vi "MGI SRS Table Settings.vi"(7 "Command":T1, 8 "Error In":errorcluster, 10 "MCLB Info In":T2, 11 "Graph/Chart Ref":refnum<vi>) -> (0 "Error Out":errorcluster, 2 "MCLB Info Out":T2)   [LabVIEW 2020]
doc: "Populates the Table Settings cluster with values from the Table of the specified Refnum.\n\nNote: Only the columns that have header strings are saved.\n\nAuthored by Shawn Walpole\nsupport@mooregoodideas.com\nwww.mooregoodideas.com\n\nCopyright (c) 2010, Moore Good Ideas, Inc.\n\nAll rights reserved.\n\nRedistribution and use in source and binary forms, with or without modification, are permitted provided that the following conditions are met:\n\n * Redistributions of source code must retain the above copyright notice, this list of conditions and the following disclaimer.\n * Redistributions in binary form must reproduce the above copyright notice, this list of conditions and the following disclaimer in the documentation and/or other materials provided with the distribution.\n * Neither the name of Moore Good Ideas, Inc. nor the names of its contributors may be used to endorse or promote products derived from this software without specific prior written permission.\n\nTHIS SOFTWARE IS PROVIDED BY THE COPYRIGHT HOLDERS AND CONTRIBUTORS \"AS IS\" AND ANY EXPRESS OR IMPLIED WARRANTIES, INCLUDING, BUT NOT LIMITED TO, THE IMPLIED WARRANTIES OF MERCHANTABILITY AND FITNESS FOR A PARTICULAR PURPOSE ARE DISCLAIMED. IN NO EVENT SHALL THE COPYRIGHT OWNER OR CONTRIBUTORS BE LIABLE FOR ANY DIRECT, INDIRECT, INCIDENTAL, SPECIAL, EXEMPLARY, OR CONSEQUENTIAL DAMAGES (INCLUDING, BUT NOT LIMITED TO, PROCUREMENT OF SUBSTITUTE GOODS OR SERVICES; LOSS OF USE, DATA, OR PROFITS; OR BUSINESS INTERRUPTION) HOWEVER CAUSED AND ON ANY THEORY OF LIABILITY, WHETHER IN CONTRACT, STRICT LIABILITY, OR TORT (INCLUDING NEGLIGENCE OR OTHERWISE) ARISING IN ANY WAY OUT OF THE USE OF THIS SOFTWARE, EVEN IF ADVISED OF THE POSSIBILITY OF SUCH DAMAGE."
uses:
  <userlib>/_MGI/Application Control/MGI Save & Restore Settings/MGI SRS Command Enum.ctl
  <userlib>/_MGI/Application Control/MGI Save & Restore Settings/MGI SRS MCLB Setting Cluster.ctl
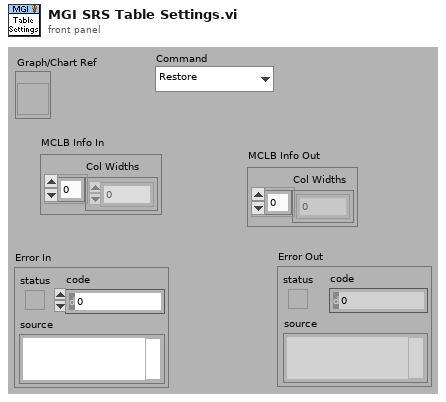
[diagram p1: front panel]
types:
  T1 = typedef "MGI SRS Command Enum.ctl" = enum16{"Restore", "Save"}
  T2 = typedef "MGI SRS MCLB Setting Cluster.ctl" = cluster{"Col Widths":i32[]}
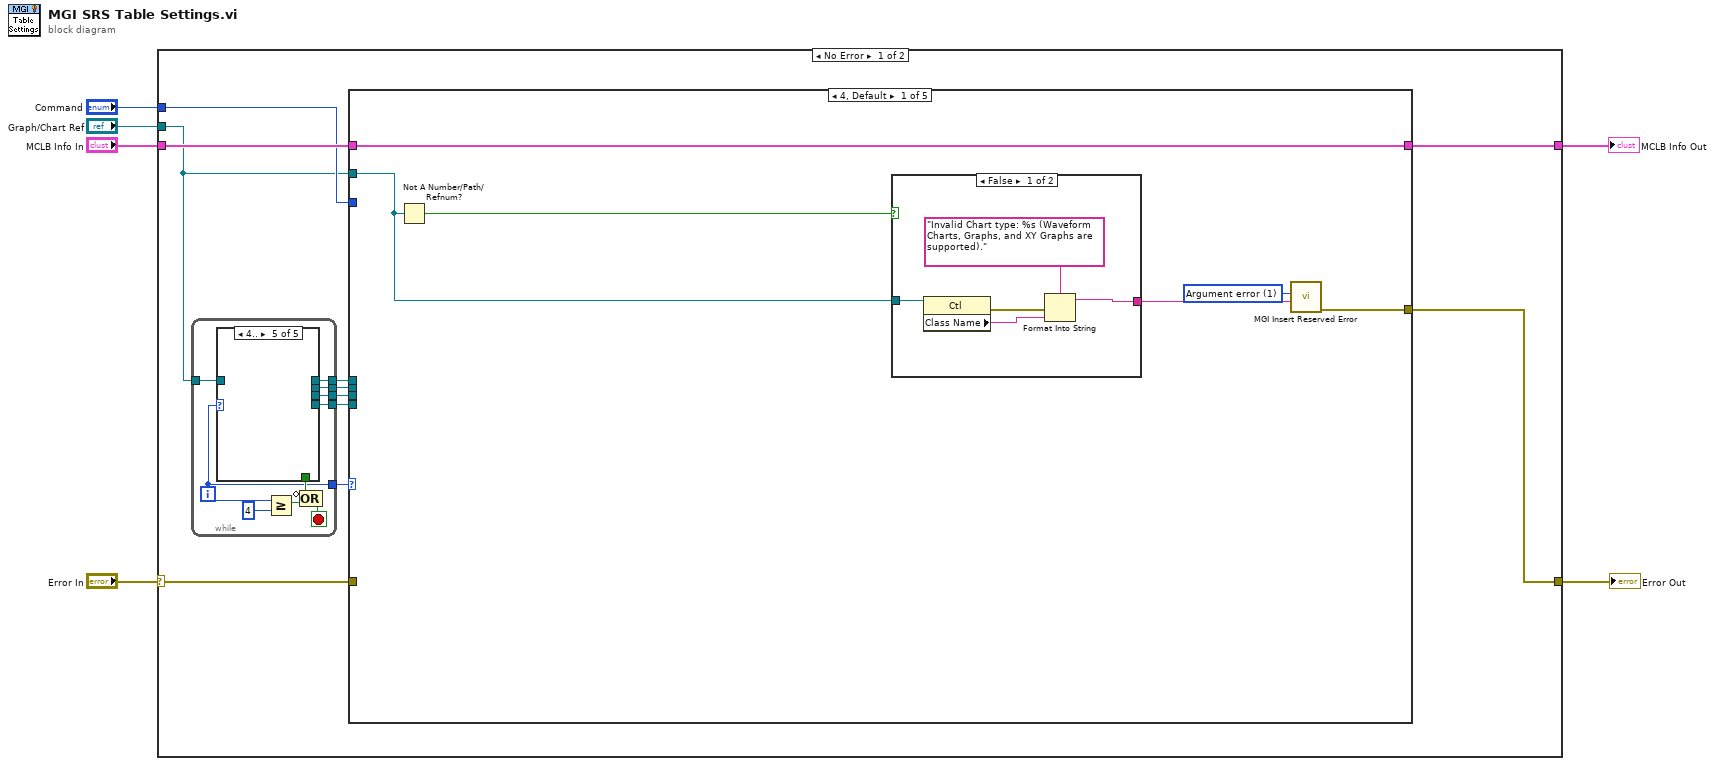
[diagram p0: block diagram]
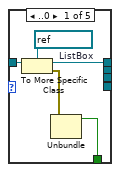
[diagram p2: hidden frame]
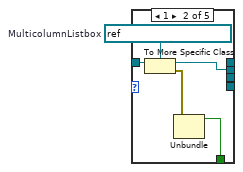
[diagram p3: hidden frame]
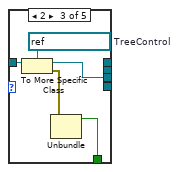
[diagram p4: hidden frame]
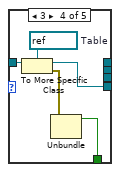
[diagram p5: hidden frame]
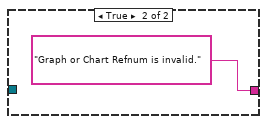
[diagram p6: hidden frame]
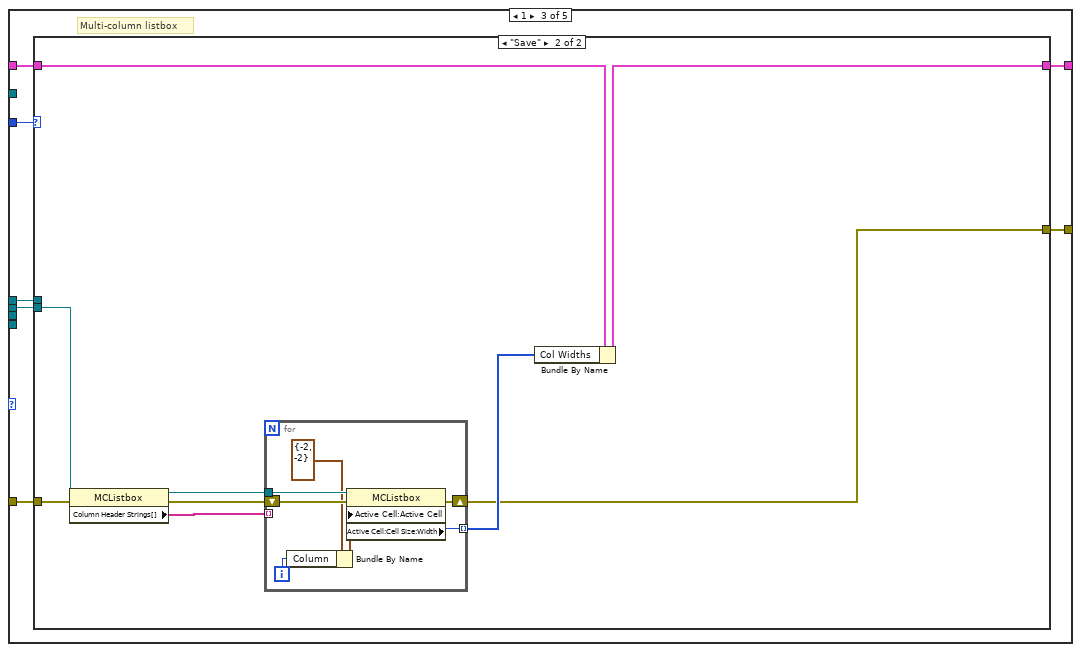
[diagram p9: hidden frame]
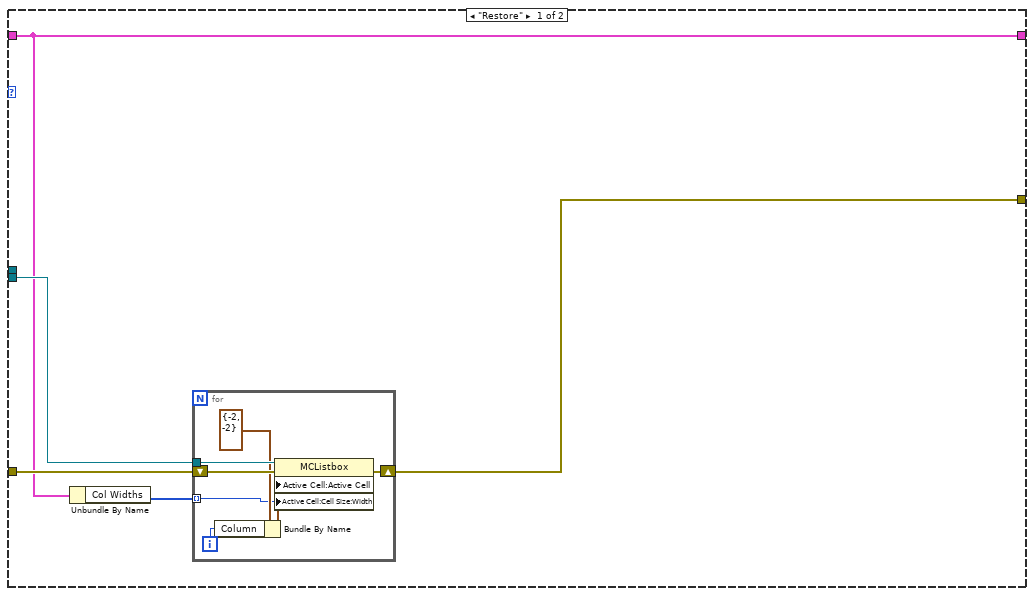
[diagram p10: hidden frame]
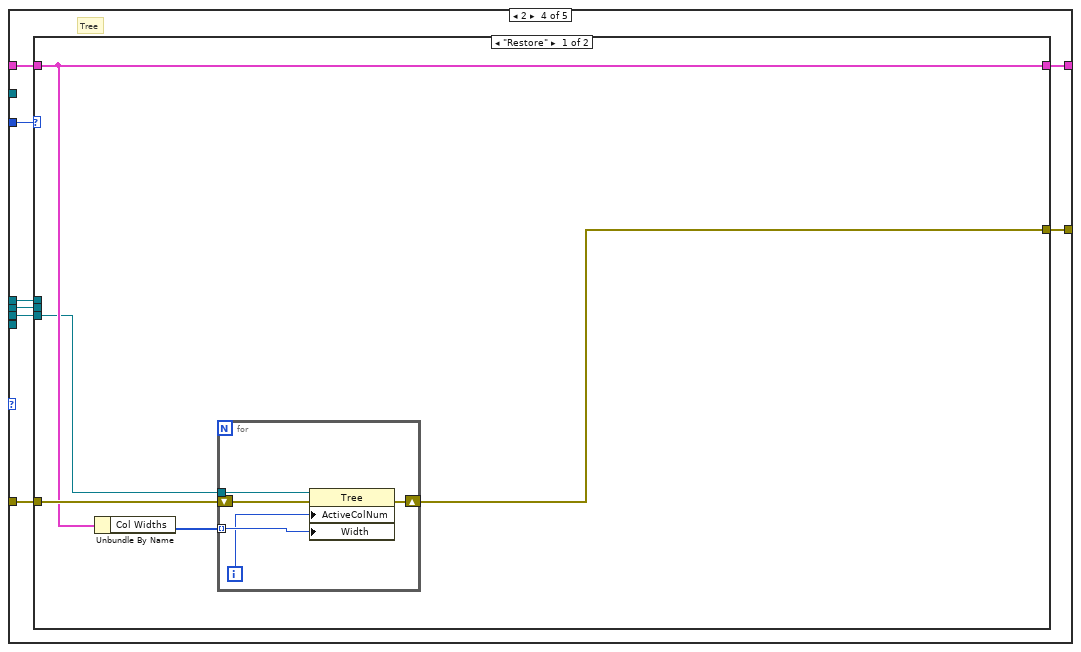
[diagram p11: hidden frame]
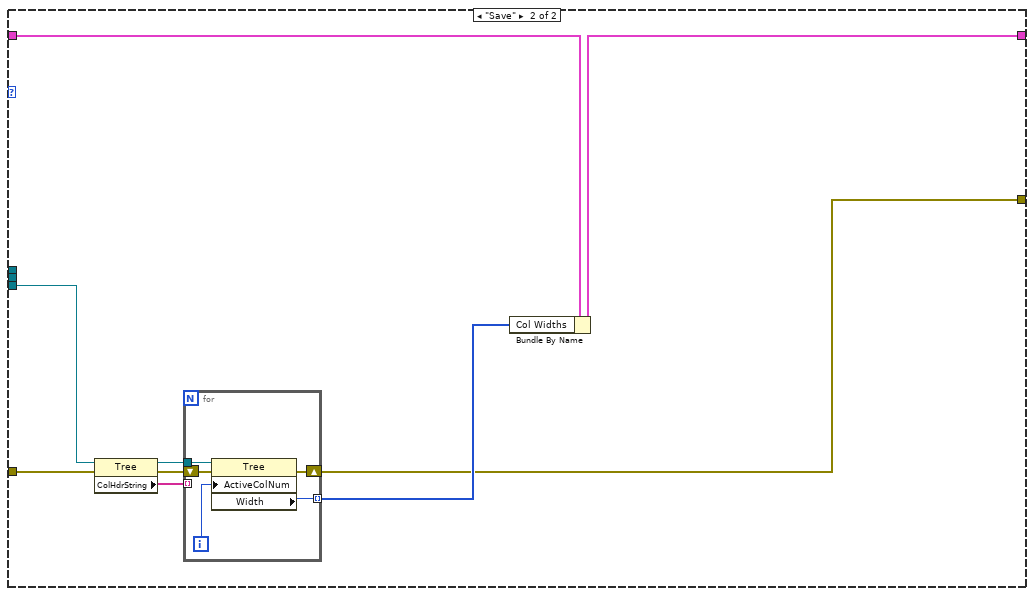
[diagram p12: hidden frame]
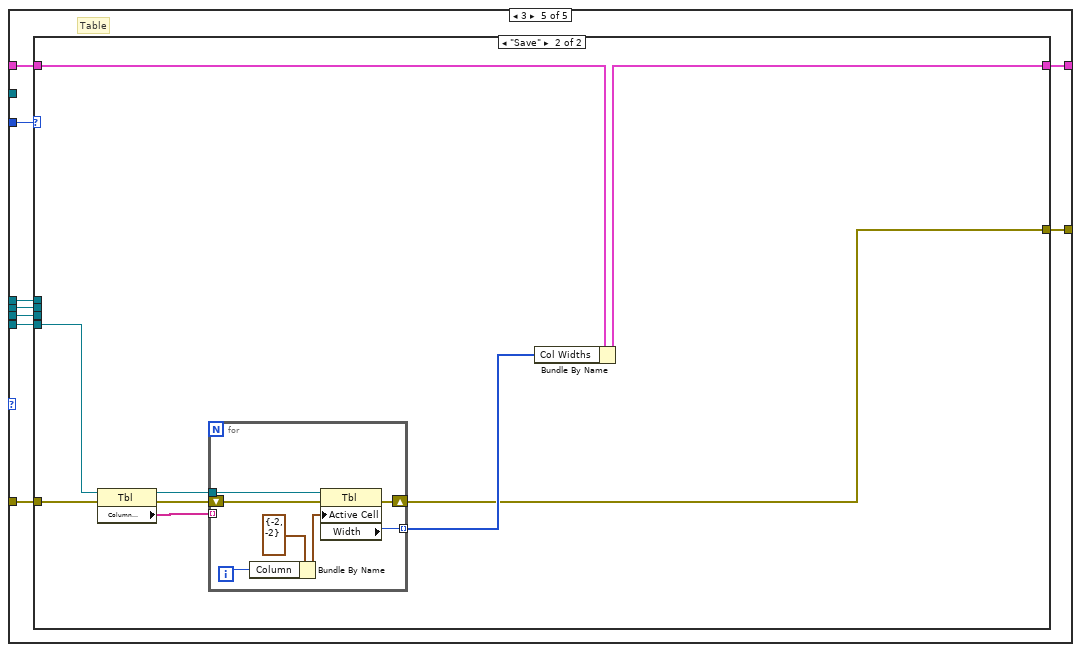
[diagram p13: hidden frame]
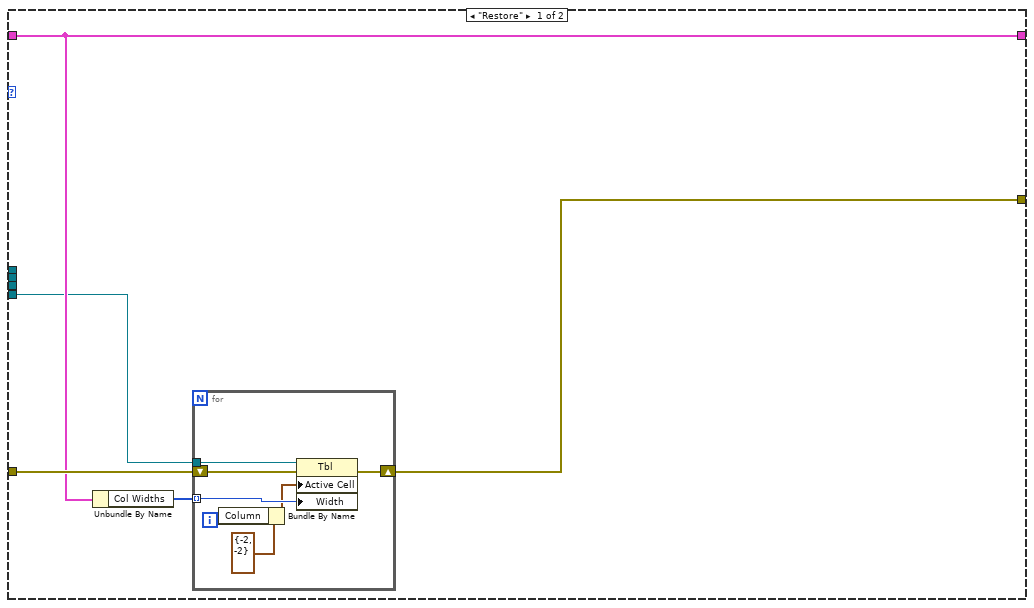
[diagram p14: hidden frame]
diagram:
  n1 = case shown="No Error" "Error In" {
    selector: "Error In" -> [w9 w175]
    tunnel: "Command" -> [w8 _]
    tunnel: "Graph/Chart Ref" -> [w7 _]
    tunnel: "MCLB Info In" -> [w17 w174]
    tunnel: [w16 w174] -> w2
    tunnel: [w15 w175] -> w1
    frame No Error {
      n2 = while {
        tunnel: w7 -> [w27]
        tunnel: [w22] -> w14
        tunnel: [w21] -> w13
        tunnel: [w20] -> w12
        tunnel: [w19] -> w11
        tunnel: [w18] -> w10
        i -> [w18]
        stop <- w24 stop-if-true
        n3 = case shown="4.." w18 {
          tunnel: w27 -> [w32 w37 w42 w47 _]
          tunnel: [w29 w34 w39 w44 _] -> w23
          tunnel: [_ _ _ w43 _] -> w22
          tunnel: [_ _ w38 _ _] -> w21
          tunnel: [_ w33 _ _ _] -> w20
          tunnel: [w28 _ _ _ _] -> w19
          frame ..0 {
            w31 = refnum<vi> refnum  # ListBox
            n4 = To More Specific Class(target class=w31, reference=w32) -> (specific class reference=w28:refnum<vi>, error out=w30:errorcluster)  [unwired: 1 in]
            n5 = Unbundle(w30) -> ("status"=w29:bool)  [unwired: 2 out]
          }
          frame 1 {
            w36 = refnum<vi> refnum  # MulticolumnListbox
            n6 = To More Specific Class(target class=w36, reference=w37) -> (specific class reference=w33:refnum<vi>, error out=w35:errorcluster)  [unwired: 1 in]
            n7 = Unbundle(w35) -> ("status"=w34:bool)  [unwired: 2 out]
          }
          frame 2 {
            w41 = refnum<vi> refnum  # TreeControl
            n8 = To More Specific Class(target class=w41, reference=w42) -> (specific class reference=w38:refnum<vi>, error out=w40:errorcluster)  [unwired: 1 in]
            n9 = Unbundle(w40) -> ("status"=w39:bool)  [unwired: 2 out]
          }
          frame 3 {
            w46 = refnum<vi> refnum  # Table
            n10 = To More Specific Class(target class=w46, reference=w47) -> (specific class reference=w43:refnum<vi>, error out=w45:errorcluster)  [unwired: 1 in]
            n11 = Unbundle(w45) -> ("status"=w44:bool)  [unwired: 2 out]
          }
          frame 4.. {
          }
        }
        n12 = Greater Or Equal?(x=w18, y=4) -> (x >= y?=w25:bool)
        n13 = Compound Arithmetic op=OR(invert w23, w25) -> (w24:bool)
      }
      n14 = case shown="4, Default" w10 {
        tunnel: [w49 w65 w76 w112 w145] -> w15
        tunnel: w7 -> [w53 _ _ _ _]
        tunnel: w17 -> [w52 w61 w72 w108 w141]
        tunnel: [w52 w60 w71 w107 w140] -> w16
        tunnel: w14 -> [_ _ _ _ w137]
        tunnel: w13 -> [_ _ _ w105 w138]
        tunnel: w12 -> [_ _ w70 w106 w139]
        tunnel: w11 -> [_ w63 w74 w110 w143]
        tunnel: w9 -> [_ w62 w73 w109 w142]
        tunnel: w8 -> [_ w64 w75 w111 w144]
        frame 4, Default {
          w50 = u16 1 items=["No error", "Argument error", "Memory is full", "Out of zone", "End of file", "File already open", "Generic file I/O error", "File not found", "File permission error", "Disk is full", "Duplicate path", "Too many files open", "System feature not enabled", "Resource file not found", "Cannot add resource", "Resource not found", "Image not found", "Image memory error", "Pen does not exist", "Config type invalid", "Config token not found", "Config parse error", "Config memory error", "Bad external code format", "Bad external code offset", "External code not present", "Null window", "Destroy window error", "Null menu", "Print aborted", "Bad print record", "Print driver error", "Windows error during printing", "Memory error during printing", "Print dialog error", "Generic print error", "Invalid device refnum", "Device not found", "Device parameter error", "Device unit error", "Cannot open device", "Device call aborted", "Generic error", "Cancelled by user", "Object ID too low", "Object ID too high", "Object not in heap", "Unknown heap", "Unknown object (invalid DefProc)", "Unknown object (DefProc not in table)", "Message out of range", "Invalid (null) method", "Unknown message", "Manager call not supported", "Bad address", "Network operation in progress", "Network operation timed out", "Connection is busy", "Network attribute not supported", "Network error", "Address in use", "System out of memory", "Connection aborted", "Connection refused", "Not connected", "Already connected", "Connection closed", "Initialization error (interapplication manager)", "Bad occurrence", "Wait on unbound occurrence handler", "Occurrence queue overflow", "Datalog type conflict", "Unused", "Unrecognized type (interapplication manager)", "Memory corrupt", "Failed to make temporary DLL", "Old CIN version", "Drag socket not found", "Failed to load drop-object", "Failed to register OLE object", "Failed to release OLE object", "Format specifier type mismatch", "Unknown format specifier", "Too few format specifiers", "Too many format specifiers", "Scan failed", "Newer CIN version", "OLE Convert", "Runtime menu error", "Password tampered", "Unknown error code"] ("Reserved Error Code (Generic error)")
          n15 = Not A Number/Path/Refnum?(number/path/refnum=w53) -> (NaN/Path/Refnum?=w51:bool)
          n16 = case shown="False" w51 {
            tunnel: [w55 "Graph or Chart Refnum is invalid." ("format string")] -> w48
            tunnel: w53 -> [w54 _]
            frame False {
              n17 = property class="Ctl"(reference=w54) -> (error out=w56:errorcluster, "Class Name"=w58:string)  [unwired: 1 in, 1 out]
              n18 = Format Into String(format string="Invalid Chart type: %s (Waveform Charts, Graphs, and XY Graphs are supported).", error in=w56, w58) -> (resulting string=w55:string)  [unwired: 1 in, 1 out]
            }
            frame True {
            }
          }
          n19 = call <userlib>:"MGI Insert Reserved Error.vi"("Error Description"=w48, "Reserved Error Code (Generic error)"=w50) -> ("Error Out"=w49:errorcluster)  [unwired: 9 in]
        }
        frame 0 {
          # "Listbox only has 1 column; nothing to do."
          n20 = case shown="\"Save\"" w64 {
            tunnel: [w66 w69] -> w65
            tunnel: w63 -> [_ _]
            tunnel: w62 -> [w66 w69]
            tunnel: w61 -> [w67 w68]
            tunnel: [w67 w68] -> w60
            frame "Restore" {
            }
            frame "Save" {
            }
          }
        }
        frame 1 {
          # "Multi-column listbox"
          n21 = case shown="\"Save\"" w75 {
            tunnel: [w77 w90] -> w76
            tunnel: w74 -> [_ _]
            tunnel: w73 -> [w81 w93]
            tunnel: w72 -> [w79 w92]
            tunnel: [w79 w89] -> w71
            tunnel: w70 -> [w80 w94]
            frame "Restore" {
              n22 = Unbundle By Name(w79) -> ("Col Widths"=w78:i32[])
              n23 = for {
                shift-right: [w86] -> w77
                shift-left: w81 -> [w87]
                tunnel: w80 -> [w88]
                tunnel: w78 -> [w82] mode=indexing
                i -> [w84]
                n24 = Bundle By Name(cluster=cluster{"Row":i32, "Column":i32} {"Row"=-2, "Column"=-2} ("Active Cell:Active Cell"), "Column"=w84) -> (w83:cluster{"Row":i32, "Column":i32})
                n25 = property class="MCListbox"(reference=w88, error in=w87, "Active Cell:Active Cell"=w83, "Active Cell:Cell Size:Width"=w82) -> (error out=w86:errorcluster)  [unwired: 1 out]
              }
            }
            frame "Save" {
              n26 = property class="MCListbox"(reference=w94, error in=w93) -> (reference out=w95:refnum<vi>, error out=w96:errorcluster, "Column Header Strings[]"=w97:string[])
              n27 = for {
                tunnel: w97 -> [_] mode=indexing
                shift-right: [w102] -> w90
                shift-left: w96 -> [w103]
                tunnel: w95 -> [w104]
                tunnel: [w101] -> w91 mode=indexing
                i -> [w99]
                n28 = Bundle By Name(cluster=cluster{"Row":i32, "Column":i32} {"Row"=-2, "Column"=-2} ("Active Cell:Active Cell"), "Column"=w99) -> (w98:cluster{"Row":i32, "Column":i32})
                n29 = property class="MCListbox"(reference=w104, error in=w103, "Active Cell:Active Cell"=w98) -> (error out=w102:errorcluster, "Active Cell:Cell Size:Width"=w101:u32)  [unwired: 1 out]
              }
              n30 = Bundle By Name(cluster=w92, "Col Widths"=w91) -> (w89:T2)
            }
          }
        }
        frame 2 {
          # "Tree"
          n31 = case shown="\"Restore\"" w111 {
            tunnel: [w114 w125] -> w112
            tunnel: w110 -> [_ _]
            tunnel: w109 -> [w117 w128]
            tunnel: w108 -> [w116 w127]
            tunnel: [w116 w124] -> w107
            tunnel: w106 -> [_ _]
            tunnel: w105 -> [w113 w123]
            frame "Restore" {
              n32 = Unbundle By Name(w116) -> ("Col Widths"=w115:i32[])
              n33 = for {
                shift-right: [w120] -> w114
                shift-left: w117 -> [w121]
                tunnel: w113 -> [w122]
                tunnel: w115 -> [w119] mode=indexing
                i -> [w118]
                n34 = property class="Tree"(reference=w122, error in=w121, "ActiveColNum"=w118, "Width"=w119) -> (error out=w120:errorcluster)  [unwired: 1 out]
              }
            }
            frame "Save" {
              n35 = property class="Tree"(reference=w123, error in=w128) -> (reference out=w129:refnum<vi>, error out=w130:errorcluster, "ColHdrString"=w131:string[])
              n36 = for {
                tunnel: w131 -> [_] mode=indexing
                shift-right: [w134] -> w125
                shift-left: w130 -> [w135]
                tunnel: w129 -> [w136]
                tunnel: [w133] -> w126 mode=indexing
                i -> [w132]
                n37 = property class="Tree"(reference=w136, error in=w135, "ActiveColNum"=w132) -> (error out=w134:errorcluster, "Width"=w133:i32)  [unwired: 1 out]
              }
              n38 = Bundle By Name(cluster=w127, "Col Widths"=w126) -> (w124:T2)
            }
          }
        }
        frame 3 {
          # "Table"
          n39 = case shown="\"Save\"" w144 {
            tunnel: [w147 w160] -> w145
            tunnel: w143 -> [_ _]
            tunnel: w142 -> [w150 w163]
            tunnel: w141 -> [w149 w162]
            tunnel: [w149 w159] -> w140
            tunnel: w139 -> [_ _]
            tunnel: w138 -> [_ _]
            tunnel: w137 -> [w146 w158]
            frame "Restore" {
              n40 = Unbundle By Name(w149) -> ("Col Widths"=w148:i32[])
              n41 = for {
                shift-right: [w155] -> w147
                shift-left: w150 -> [w156]
                tunnel: w146 -> [w157]
                tunnel: w148 -> [w154] mode=indexing
                i -> [w152]
                n42 = Bundle By Name(cluster=cluster{"Row":i32, "Column":i32} {"Row"=-2, "Column"=-2} ("Active Cell:Active Cell"), "Column"=w152) -> (w151:cluster{"Row":i32, "Column":i32})
                n43 = property class="Tbl"(reference=w157, error in=w156, "Active Cell"=w151, "Width"=w154) -> (error out=w155:errorcluster)  [unwired: 1 out]
              }
            }
            frame "Save" {
              n44 = property class="Tbl"(reference=w158, error in=w163) -> (reference out=w164:refnum<vi>, error out=w165:errorcluster, "Column Headers[]"=w166:string[])
              n45 = for {
                tunnel: w166 -> [_] mode=indexing
                shift-right: [w172] -> w160
                shift-left: w165 -> [w167]
                tunnel: w164 -> [w173]
                tunnel: [w171] -> w161 mode=indexing
                i -> [w169]
                n46 = Bundle By Name(cluster=cluster{"Row":i32, "Column":i32} {"Row"=-2, "Column"=-2} ("Active Cell:Active Cell"), "Column"=w169) -> (w168:cluster{"Row":i32, "Column":i32})
                n47 = property class="Tbl"(reference=w173, error in=w167, "Active Cell"=w168) -> (error out=w172:errorcluster, "Width"=w171:u32)  [unwired: 1 out]
              }
              n48 = Bundle By Name(cluster=w162, "Col Widths"=w161) -> (w159:T2)
            }
          }
        }
      }
    }
    frame Error {
    }
  }
  "MCLB Info Out" <- w2
  "Error Out" <- w1
